vi "pp2_log_error.vi"(6 "error in (no error)":errorcluster, 9 "queue in":refnum<queue>) -> (0 "error out":errorcluster, 3 "queue out":refnum<queue>)   [LabVIEW 2013]
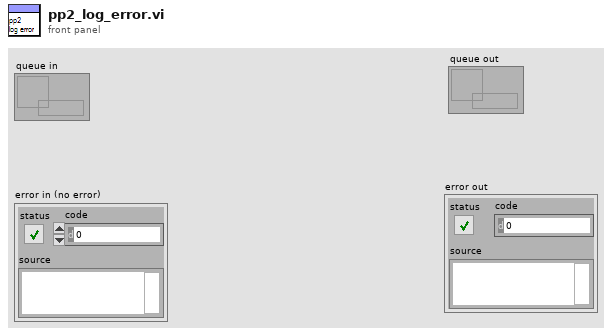
[diagram p1: front panel]
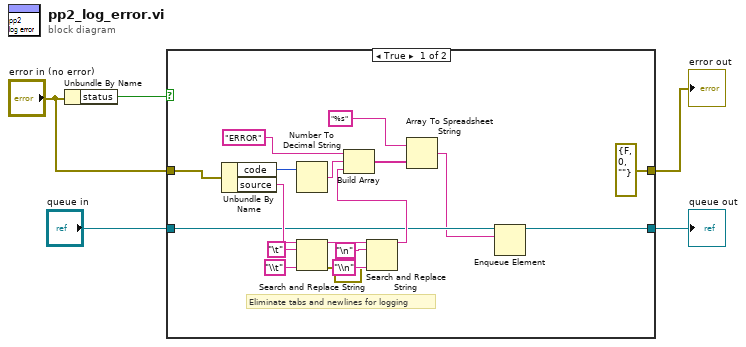
[diagram p0: block diagram]
diagram:
  n1 = Unbundle By Name("error in (no error)") -> ("status"=w5:bool)
  n2 = case shown="True" w5 {
    tunnel: "error in (no error)" -> [w23 w24]
    tunnel: "queue in" -> [w8 w25]
    tunnel: [w7 w25] -> w1
    tunnel: [errorcluster {"status"=FALSE, "code"=0, "source"=""} ("error in (no error)") w24] -> w3
    frame True {
      # "Eliminate tabs and newlines for logging"
      n3 = Unbundle By Name(w23) -> ("code"=w21:i32, "source"=w16:string)
      n4 = Number To Decimal String(number=w21) -> (decimal integer string=w20:string)  [unwired: 1 in]
      n5 = Search and Replace String(input string=w16, search string="\t", replace string="\\t" ("replace string (\"\")")) -> (result string=w11:string, error out=w10:errorcluster)  [unwired: 5 in, 2 out]
      n6 = Search and Replace String(input string=w11, search string="\n", replace string="\\n" ("replace string (\"\")"), error in=w10) -> (result string=w9:string)  [unwired: 4 in, 3 out]
      n7 = Build Array("ERROR" ("element"), w20, w9) -> (w18:string[])
      n8 = Array To Spreadsheet String(array=w18, 3:"%s" ("format string")) -> (spreadsheet string=w6:string)  [unwired: 1 in]
      n9 = Enqueue Element(queue=w8, element=w6) -> (queue out=w7:refnum<queue>)  [unwired: 2 in, 2 out]
    }
    frame False {
    }
  }
  "error out" <- w3
  "queue out" <- w1
